vi "Test Steer Jaguars.vi"   [LabVIEW 2011]
types:
  T1 = typedef "WPI_MotorControlDeviceRef.ctl" = cluster{"DeviceStatus":errorcluster, "Type":enum16{"PWM", "CAN"}, "PWM":cluster{"Digital Module":T2, "PWM Channel":T3, "DeadBand":T4}, "CAN":cluster{"Device Number":u8, "Control Mode":T5, "Semaphore":T6, "Max Vout":dbl}, "Invert":bool, "TransformRef":T7, "InvTransformRef":T7}
  T2 = typedef "FPGA_TypedefDigitalModule.ctl" = enum16{"Digital Module 1", "Digital Module 2"}
  T3 = typedef "FPGA_DIOPWMChannel.ctl" = enum8{"PWM 1", "PWM 2", "PWM 3", "PWM 4", "PWM 5", "PWM 6", "PWM 7", "PWM 8", "PWM 9", "PWM 10", "Invalid"}
  T4 = typedef "WPI_PWMDeadband.ctl" = cluster{"Name":string, "maxPositivePwm":i32, "minPositivePwm":i32, "centerPwm":i32, "maxNegativePwm":i32, "minNegativePwm":i32, "angularRange":u16}
  T5 = typedef "WPI_CANJaguar_ControlMode.ctl" = enum8{"Percent VBus", "Current", "Speed", "Position", "Voltage"}
  T6 = typedef "Semaphore RefNum" = refnum<k1>
  T7 = typedef "WPI_PWMTransform_ConPane.ctl" = refnum<vi>
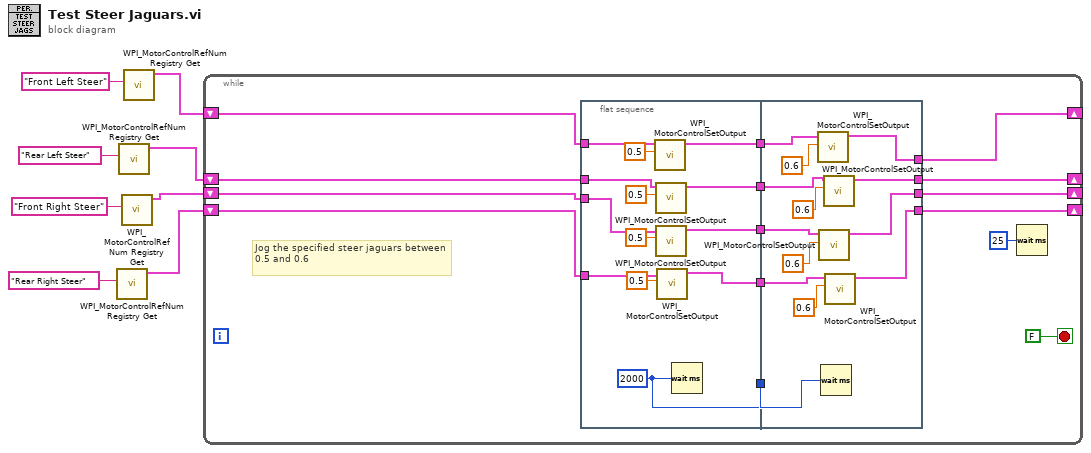
[diagram p0: block diagram]
diagram:
  n1 = call <vilib>:"WPI_MotorControlRefNum Registry Get.vi"("refnum name"="Rear Right Steer") -> ("MotorControlDevRef"=w8:T1)  [unwired: 9 in, 1 out]
  n2 = call <vilib>:"WPI_MotorControlRefNum Registry Get.vi"("refnum name"="Rear Left Steer") -> ("MotorControlDevRef"=w4:T1)  [unwired: 9 in, 1 out]
  n3 = call <vilib>:"WPI_MotorControlRefNum Registry Get.vi"("refnum name"="Front Right Steer") -> ("MotorControlDevRef"=w7:T1)  [unwired: 9 in, 1 out]
  n4 = call <vilib>:"WPI_MotorControlRefNum Registry Get.vi"("refnum name"="Front Left Steer") -> ("MotorControlDevRef"=w3:T1)  [unwired: 9 in, 1 out]
  n5 = while {
    shift-right: [w23] -> _
    shift-left: w4 -> [w19]
    shift-right: [w16] -> _
    shift-left: w3 -> [w15]
    shift-right: [w12] -> _
    shift-left: w7 -> [w14]
    shift-right: [w9] -> _
    shift-left: w8 -> [w11]
    stop <- FALSE stop-if-true
    # "Jog the specified steer jaguars between 0.5 and 0.6"
    n6 = flat-sequence {
      tunnel: [w36] -> w21
      tunnel: [w35] -> w20
      tunnel: w19 -> [w33]
      tunnel: w15 -> [w31]
      tunnel: [w30] -> w17
      tunnel: w14 -> [w27]
      tunnel: [w26] -> w13
      tunnel: w11 -> [w25]
      tunnel: [w24] -> w10
      tunnel: w21 -> [w49]
      tunnel: [w48] -> w23
      tunnel: w20 -> [w47]
      tunnel: w17 -> [w44]
      tunnel: [w43] -> w16
      tunnel: w13 -> [w40]
      tunnel: [w39] -> w12
      tunnel: w10 -> [w38]
      tunnel: [w37] -> w9
      frame #0 {
        w35 = u32 2000 ("milliseconds to wait")
        n7 = call <vilib>:"WPI_MotorControlSetOutput.vi"("Output"=0.5, "MotorControlDevRef"=w31) -> ("MotorControlDevRef"=w30:T1)  [unwired: 8 in, 1 out]
        n8 = call <vilib>:"WPI_MotorControlSetOutput.vi"("Output"=0.5, "MotorControlDevRef"=w33) -> ("MotorControlDevRef"=w36:T1)  [unwired: 8 in, 1 out]
        n9 = call <vilib>:"WPI_MotorControlSetOutput.vi"("Output"=0.5, "MotorControlDevRef"=w27) -> ("MotorControlDevRef"=w26:T1)  [unwired: 8 in, 1 out]
        n10 = call <vilib>:"WPI_MotorControlSetOutput.vi"("Output"=0.5, "MotorControlDevRef"=w25) -> ("MotorControlDevRef"=w24:T1)  [unwired: 8 in, 1 out]
        n11 = Wait (ms)(milliseconds to wait=w35) -> ()  [unwired: 1 out]
      }
      frame #1 {
        n12 = call <vilib>:"WPI_MotorControlSetOutput.vi"("Output"=0.6, "MotorControlDevRef"=w44) -> ("MotorControlDevRef"=w43:T1)  [unwired: 8 in, 1 out]
        n13 = call <vilib>:"WPI_MotorControlSetOutput.vi"("Output"=0.6, "MotorControlDevRef"=w40) -> ("MotorControlDevRef"=w39:T1)  [unwired: 8 in, 1 out]
        n14 = Wait (ms)(milliseconds to wait=w47) -> ()  [unwired: 1 out]
        n15 = call <vilib>:"WPI_MotorControlSetOutput.vi"("Output"=0.6, "MotorControlDevRef"=w49) -> ("MotorControlDevRef"=w48:T1)  [unwired: 8 in, 1 out]
        n16 = call <vilib>:"WPI_MotorControlSetOutput.vi"("Output"=0.6, "MotorControlDevRef"=w38) -> ("MotorControlDevRef"=w37:T1)  [unwired: 8 in, 1 out]
      }
    }
    n17 = Wait (ms)(milliseconds to wait=u32 25) -> ()  [unwired: 1 out]
  }
